vi "ZwangsbedingungenGV_ECD.vi"(4 "AnzahlHorst":i32, 5 "AnzahlHorst/Modul":i32[](array[numeric]), 6 "AnzahlLH":i32, 7 "AnzahlDIOs/Modul":i32[](array[numeric]), 8 "AnzahlDIOs":i32, 9 "Zwangsbedingungen":dbl[][](array[numeric]), 10 "Methodennummer":i32(ring) items=["0"]) -> (1 "Methodennummer":i32(ring) items=["0"])   [LabVIEW 2017]
uses:
  GVMWHorst_ECD.vi
  GVHK1Hz_ECD.vi
  gvbooleschRT_ECD.vi
  GVZeitenZyklen_ECD.vi
  GVVentilposition_ECD.vi
  GVMetavariablen_ECD.vi
  GVZwangs_ECD.vi
  GVZwangsMPVPos_ECD.vi
  GVZwangsMPV_ECD.vi
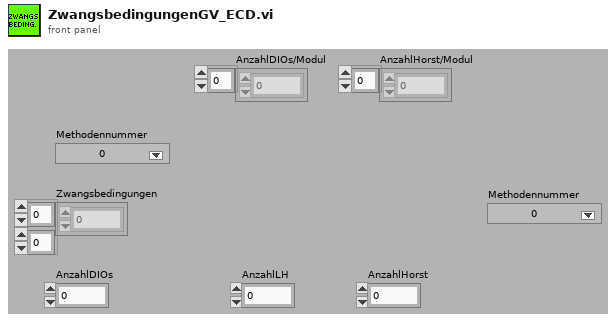
[diagram p1: front panel]
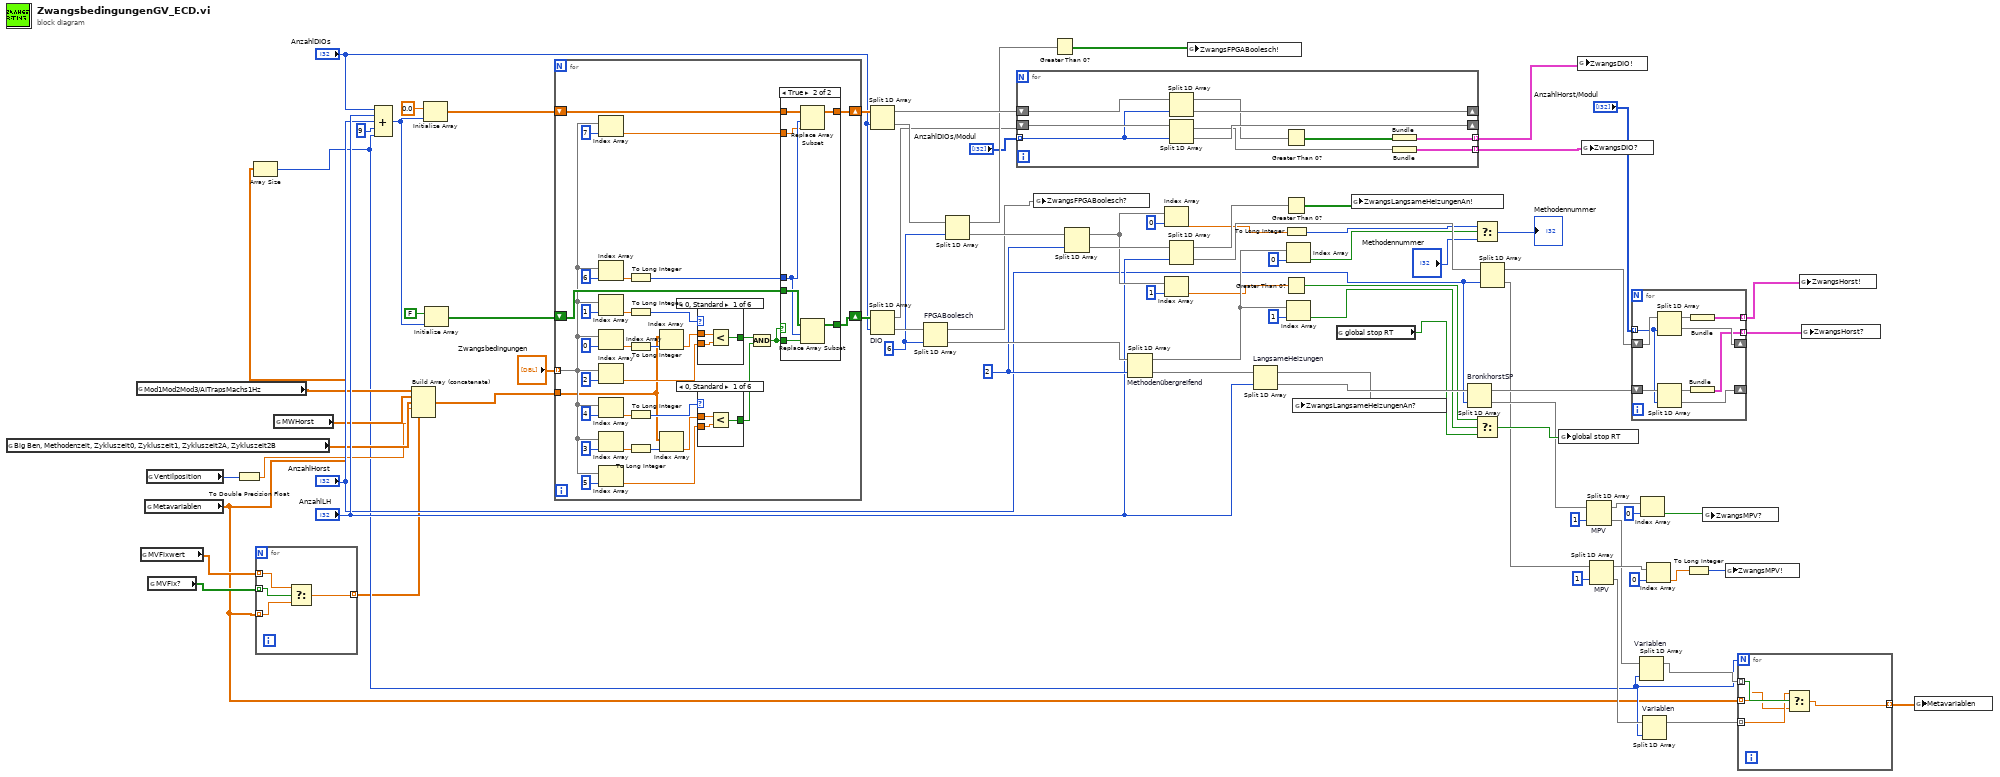
[diagram p0: block diagram]
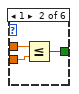
[diagram p2: hidden frame]
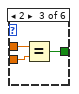
[diagram p3: hidden frame]
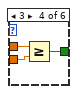
[diagram p4: hidden frame]
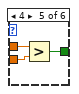
[diagram p5: hidden frame]
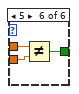
[diagram p6: hidden frame]
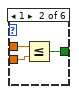
[diagram p8: hidden frame]
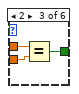
[diagram p9: hidden frame]
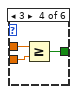
[diagram p10: hidden frame]
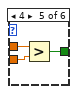
[diagram p11: hidden frame]
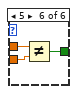
[diagram p12: hidden frame]
diagram:
  w64 = 2 ("Index")
  w74 = 6 ("Index")
  n1 = global read "GVZeitenZyklen_ECD.vi" "Big Ben, Methodenzeit, Zykluszeit0, Zykluszeit1, Zykluszeit2A, Zykluszeit2B"() -> (w24:dbl[])
  n2 = global read "GVHK1Hz_ECD.vi" "Mod1Mod2Mod3/AITrapsMachs1Hz"() -> (w27:dbl[])
  n3 = global read "GVMetavariablen_ECD.vi" "MVFixwert"() -> (w3:dbl[])
  n4 = global read "GVMetavariablen_ECD.vi" "Metavariablen"() -> (w2:dbl[])
  n5 = global read "GVVentilposition_ECD.vi" "Ventilposition"() -> (w23:i32)
  n6 = global read "GVMetavariablen_ECD.vi" "MVFix?"() -> (w4:bool[])
  n7 = To Double Precision Float(number=w23) -> (double precision float=w22:dbl)
  n8 = Array Size(array=w2) -> (size(s)=w5:i32)
  n9 = for {
    tunnel: w4 -> [w85] mode=indexing
    tunnel: w3 -> [w84] mode=indexing
    tunnel: w2 -> [w83] mode=indexing
    tunnel: [w82] -> w1 mode=indexing
    n10 = Select(t=w84, s=w85, f=w83) -> (s? t:f=w82:dbl)
  }
  n11 = global read "GVMWHorst_ECD.vi" "MWHorst"() -> (w36:dbl[])
  n12 = Compound Arithmetic op=ADD("AnzahlDIOs", "AnzahlLH", "AnzahlHorst", 9 ("Wert"), w5) -> (w52:i32)
  n13 = Build Array (concatenate)(w27, w36, w24, w22, w1) -> (w81:dbl[])
  n14 = Initialize Array(0.0, w52) -> (w49:dbl[])
  n15 = Initialize Array(FALSE, w52) -> (w48:bool[])
  n16 = for {
    tunnel: w81 -> [w92]
    tunnel: "Zwangsbedingungen" -> [w96] mode=indexing
    shift-right: [w100] -> w80
    shift-left: w48 -> [w105]
    shift-right: [w101] -> w76
    shift-left: w49 -> [w104]
    n17 = Index Array(array=w96, index=7 ("Index")) -> (element=w102:dbl)
    n18 = Index Array(array=w96, index=6 ("Index")) -> (element=w107:dbl)
    n19 = Index Array(array=w96, index=1 ("Index")) -> (element=w114:dbl)
    n20 = Index Array(array=w96, index=0 ("Index")) -> (element=w116:dbl)
    n21 = Index Array(array=w96, index=2 ("Index")) -> (element=w110:dbl)
    n22 = Index Array(array=w96, index=4 ("Index")) -> (element=w90:dbl)
    n23 = Index Array(array=w96, index=3 ("Index")) -> (element=w91:dbl)
    n24 = Index Array(array=w96, index=5 ("Index")) -> (element=w89:dbl)
    n25 = To Long Integer(number=w107) -> (32bit integer=w103:i32)
    n26 = To Long Integer(number=w114) -> (32bit integer=w113:i32)
    n27 = To Long Integer(number=w116) -> (32bit integer=w109:i32)
    n28 = To Long Integer(number=w90) -> (32bit integer=w95:i32)
    n29 = To Long Integer(number=w91) -> (32bit integer=w93:i32)
    n30 = Index Array(array=w92, index=w109) -> (element=w112:dbl)
    n31 = Index Array(array=w92, index=w93) -> (element=w94:dbl)
    n32 = case shown="0, Standard" w113 {
      tunnel: w112 -> [w147 w149 w153 w156 w159 w162]
      tunnel: w110 -> [w146 w150 w152 w155 w158 w161]
      tunnel: [w145 w148 w151 w154 w157 w160] -> w87
      frame 0, Default {
        n33 = Less?(x=w147, y=w146) -> (x < y?=w145:bool)
      }
      frame 1 {
        n34 = Less Or Equal?(x=w149, y=w150) -> (x <= y?=w148:bool)
      }
      frame 2 {
        n35 = Equal?(x=w153, y=w152) -> (x = y?=w151:bool)
      }
      frame 3 {
        n36 = Greater Or Equal?(x=w156, y=w155) -> (x >= y?=w154:bool)
      }
      frame 4 {
        n37 = Greater?(x=w159, y=w158) -> (0:w157:bool)
      }
      frame 5 {
        n38 = Not Equal?(x=w162, y=w161) -> (x != y?=w160:bool)
      }
    }
    n39 = case shown="0, Standard" w95 {
      tunnel: w94 -> [w120 w122 w126 w129 w132 w135]
      tunnel: w89 -> [w119 w123 w125 w128 w131 w134]
      tunnel: [w118 w121 w124 w127 w130 w133] -> w88
      frame 0, Default {
        n40 = Less?(x=w120, y=w119) -> (x < y?=w118:bool)
      }
      frame 1 {
        n41 = Less Or Equal?(x=w122, y=w123) -> (x <= y?=w121:bool)
      }
      frame 2 {
        n42 = Equal?(x=w126, y=w125) -> (x = y?=w124:bool)
      }
      frame 3 {
        n43 = Greater Or Equal?(x=w129, y=w128) -> (x >= y?=w127:bool)
      }
      frame 4 {
        n44 = Greater?(x=w132, y=w131) -> (0:w130:bool)
      }
      frame 5 {
        n45 = Not Equal?(x=w135, y=w134) -> (x != y?=w133:bool)
      }
    }
    n46 = And(x=w87, y=w88) -> (x .and. y?=w86:bool)
    n47 = case shown="True" w86 {
      tunnel: w105 -> [w137 w144]
      tunnel: w104 -> [w136 w143]
      tunnel: w103 -> [_ w142]
      tunnel: w86 -> [_ w141]
      tunnel: w102 -> [_ w140]
      tunnel: [w136 w139] -> w101
      tunnel: [w137 w138] -> w100
      frame False {
      }
      frame True {
        n48 = Replace Array Subset(array=w143, new element=w140, index=w142) -> (w139:dbl[])
        n49 = Replace Array Subset(array=w144, new element=w141, index=w142) -> (w138:bool[])
      }
    }
  }
  n50 = Split 1D Array ("DIO")(array=w76, index="AnzahlDIOs") -> (first subarray=w75:dbl[], second subarray=w73:dbl[])
  n51 = Split 1D Array "DIO"(array=w80, index="AnzahlDIOs") -> (first subarray=w59:bool[], second subarray=w79:bool[])
  n52 = Split 1D Array "FPGABoolesch"(array=w79, index=w74) -> (first subarray=w35:bool[], second subarray=w68:bool[])
  n53 = Split 1D Array(array=w73, index=w74) -> (first subarray=w72:dbl[], second subarray=w66:dbl[])
  n54 = for {
    tunnel: [w165] -> w30 mode=indexing
    tunnel: "AnzahlDIOs/Modul" -> [w167] mode=indexing
    tunnel: [w163] -> w31 mode=indexing
    shift-right: [w171] -> _
    shift-left: w59 -> [w172]
    shift-right: [w169] -> _
    shift-left: w75 -> [w170]
    n55 = Split 1D Array(array=w170, index=w167) -> (first subarray=w168:dbl[], second subarray=w169:dbl[])
    n56 = Split 1D Array(array=w172, index=w167) -> (first subarray=w166:bool[], second subarray=w171:bool[])
    n57 = Greater Than 0?(x=w168) -> (x > 0?=w164:bool[])
    n58 = Bundle(w164) -> (w163:cluster{bool[]})  [unwired: 1 in]
    n59 = Bundle(w166) -> (w165:cluster{bool[]})  [unwired: 1 in]
  }
  n60 = global write "GVZwangs_ECD.vi" "ZwangsFPGABoolesch?"(w35) -> ()
  n61 = Greater Than 0?(x=w72) -> (x > 0?=w34:bool[])
  n62 = Split 1D Array(array=w66, index=w64) -> (first subarray=w60:dbl[], second subarray=w65:dbl[])
  n63 = Split 1D Array "Methodenübergreifend"(array=w68, index=w64) -> (first subarray=w62:bool[], second subarray=w67:bool[])
  n64 = Index Array(array=w60, index=0 ("Index")) -> (element=w41:dbl)
  n65 = Index Array(array=w60, index=1 ("Index")) -> (element=w45:dbl)
  n66 = Split 1D Array(array=w65, index="AnzahlLH") -> (first subarray=w69:dbl[], second subarray=w71:dbl[])
  n67 = global write "GVZwangs_ECD.vi" "ZwangsFPGABoolesch!"(w34) -> ()
  n68 = Split 1D Array "LangsameHeizungen"(array=w67, index="AnzahlLH") -> (first subarray=w33:bool[], second subarray=w78:bool[])
  n69 = Greater Than 0?(x=w69) -> (x > 0?=w32:bool[])
  n70 = To Long Integer(number=w41) -> (32bit integer=w39:i32)
  n71 = Greater Than 0?(x=w45) -> (x > 0?=w43:bool)
  n72 = Index Array(array=w62, index=0 ("Index")) -> (element=w40:bool)
  n73 = Index Array(array=w62, index=1 ("Index")) -> (element=w44:bool)
  n74 = global write "GVZwangs_ECD.vi" "ZwangsLangsameHeizungenAn?"(w33) -> ()
  n75 = global read "gvbooleschRT_ECD.vi" "global stop RT"() -> (w26:bool)
  n76 = global write "GVZwangs_ECD.vi" "ZwangsLangsameHeizungenAn!"(w32) -> ()
  n77 = Split 1D Array "BronkhorstSP"(array=w78, index="AnzahlHorst") -> (first subarray=w77:bool[], second subarray=w21:bool[])
  n78 = Select(t=w39, s=w40, f="Methodennummer") -> (s? t:f=→"Methodennummer":i32)
  n79 = Select(t=w43, s=w44, f=w26) -> (s? t:f=w25:bool)
  n80 = Split 1D Array(array=w71, index="AnzahlHorst") -> (first subarray=w70:dbl[], second subarray=w18:dbl[])
  n81 = global write "gvbooleschRT_ECD.vi" "global stop RT"(w25) -> ()
  n82 = global write "GVZwangs_ECD.vi" "ZwangsDIO!"(w31) -> ()
  n83 = global write "GVZwangs_ECD.vi" "ZwangsDIO?"(w30) -> ()
  n84 = Split 1D Array "MPV"(array=w21, index=1 ("Index")) -> (first subarray=w17:bool[], second subarray=w10:bool[])
  n85 = Split 1D Array "MPV"(array=w18, index=1 ("Index")) -> (first subarray=w13:dbl[], second subarray=w9:dbl[])
  n86 = for {
    tunnel: "AnzahlHorst/Modul" -> [w178] mode=indexing
    shift-right: [w180] -> _
    shift-left: w77 -> [w181]
    tunnel: [w175] -> w28 mode=indexing
    shift-right: [w177] -> _
    shift-left: w70 -> [w179]
    tunnel: [w173] -> w29 mode=indexing
    n87 = Split 1D Array(array=w179, index=w178) -> (first subarray=w174:dbl[], second subarray=w177:dbl[])
    n88 = Split 1D Array(array=w181, index=w178) -> (first subarray=w176:bool[], second subarray=w180:bool[])
    n89 = Bundle(w174) -> (w173:cluster{dbl[]})  [unwired: 1 in]
    n90 = Bundle(w176) -> (w175:cluster{bool[]})  [unwired: 1 in]
  }
  n91 = Split 1D Array "Variablen"(array=w10, index=w5) -> (first subarray=w8:bool[])  [unwired: 1 out]
  n92 = Index Array(array=w17, index=0 ("Index")) -> (element=w15:bool)
  n93 = Split 1D Array "Variablen"(array=w9, index=w5) -> (first subarray=w7:dbl[])  [unwired: 1 out]
  n94 = Index Array(array=w13, index=0 ("Index")) -> (element=w12:dbl)
  n95 = To Long Integer(number=w12) -> (32bit integer=w11:i32)
  n96 = global write "GVZwangsMPV_ECD.vi" "ZwangsMPV?"(w15) -> ()
  n97 = global write "GVZwangsMPVPos_ECD.vi" "ZwangsMPV!"(w11) -> ()
  n98 = for {
    N: w5 -> [_]
    tunnel: w8 -> [w185] mode=indexing
    tunnel: w7 -> [w184] mode=indexing
    tunnel: w2 -> [w183] mode=indexing
    tunnel: [w182] -> w6 mode=indexing
    n99 = Select(t=w184, s=w185, f=w183) -> (s? t:f=w182:dbl)
  }
  n100 = global write "GVZwangs_ECD.vi" "ZwangsHorst!"(w29) -> ()
  n101 = global write "GVZwangs_ECD.vi" "ZwangsHorst?"(w28) -> ()
  n102 = global write "GVMetavariablen_ECD.vi" "Metavariablen"(w6) -> ()
